vi "WriteBits.vi"(0 "Handle In":u64[](array[numeric]), 1 "error in (no error)":errorcluster, 5 "Device ID":u8=1, 7 "Write Start":u16=1, 9 "Write Amount":u16=16, 11 "WR Data":u8[](array[numeric])) -> (3 "error out":errorcluster, 4 "Handle Out":u64[](array[numeric]), 6 "Result":i32)   [LabVIEW 2020, in "SnapMB.lvlib"]
uses:
  SnapMB.lvlib
  windows/snapmb.dll
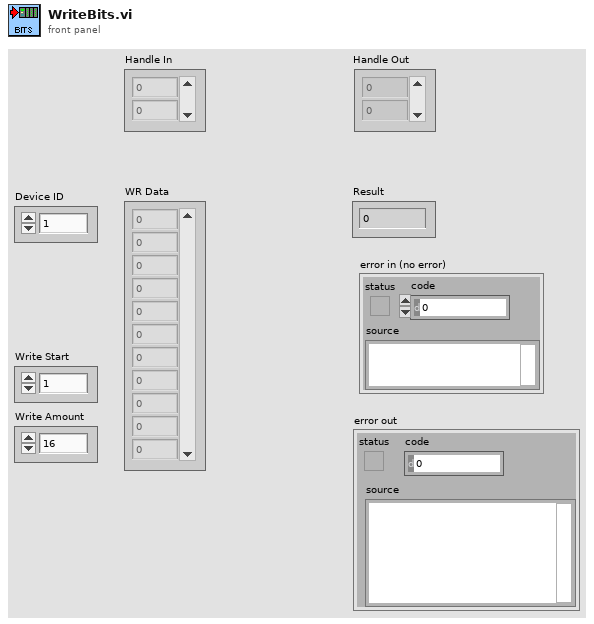
[diagram p1: front panel]
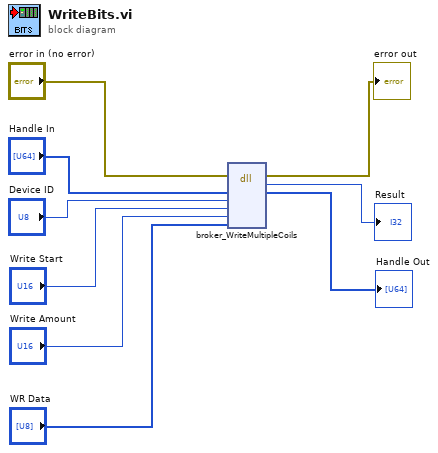
[diagram p0: block diagram]
diagram:
  n1 = dll-call lib="D:/SnapMB/LabView/lib/windows/snapmb.dll" fn="broker_WriteMultipleCoils"(error in="error in (no error)", "Handle"="Handle In", "DeviceID"="Device ID", "Start"="Write Start", "Amount"="Write Amount", "pUsrData"="WR Data") -> (error out=→"error out":errorcluster, "Result"=→"Result":i32, "Handle"=→"Handle Out":u64[])  [unwired: 6 in, 1 out]
